vi "File_Module.vi"(7 "Command":T2, 8 "error in (no error)":errorcluster, 9 "DATOS":T1={"TIEMPO"=1.0, "sFSET1"=1.0, "sFLUJO1"=1.0, "sFSET2"=0.0, "sFLUJO2"=0.0, "sFSET3"=0.0, "sFLUJO3"=0.0, "sFSET4"=0.0, "sFLUJO4"=0.0, "TSET_SUP"=0.0, "TEMP_SUP"=0.0, "TSET_INF"=0.0, "TEMP_INF"=0.0, "TSET_CINTA"=0.0, "T_CINTA"=0.0, "TSET_EXTRA"=0.0, "T_EXTRA"=0.0, "TEMP_TB"=0.0, "PESO_TB"=0.0, "POSICION"=0.0, "V_VAPOR"=0.0, "fFSET1"=0.0, "fFLUJO1"=0.0, "fFSET2"=0.0, "fFLUJO2"=0.0, "fFSET3"=0.0, "fFLUJO3"=0.0, "fFSET4"=0.0, "fFLUJO4"=0.0} {"fFSET4" format="%.2g"; "fFSET3" format="%.2g"; "fFSET2" format="%.2g"; "fFSET1" format="%.2g"; "fFLUJO4" format="%.2g"; "fFLUJO2" format="%.2g"; "fFLUJO1" format="%.2g"; "fFLUJO3" format="%.2g"; "T_EXTRA" format="%.2g"; "TSET_EXTRA" format="%.2g"; "T_CINTA" format="%.2g"; "TSET_CINTA" format="%.2g"; "sFSET4" format="%.2g"; "POSICION" format="%.2g"; "TEMP_SUP" format="%.2g"; "TSET_SUP" format="%.2g"; "PESO_TB" format="%.2g"; "TEMP_TB" format="%.2g"; "TEMP_INF" format="%.2g"; "sFSET3" format="%.2g"; "sFSET2" format="%.2g"; "sFSET1" format="%.2g"; "V_VAPOR" format="%.2g"; "sFLUJO4" format="%.2g"; "sFLUJO2" format="%.2g"; "sFLUJO1" format="%.2g"; "TSET_INF" format="%.2g"; "TIEMPO" format="%.2g"; "sFLUJO3" format="%.2g"}, 11 "Comments":string) -> (0 "error out":errorcluster, 2 "selected path":path)   [LabVIEW 2013]
uses:
  File_Module Control.ctl
  Controles/P2022 Datos Control.ctl
  P2022 TB INCAR GLOBALES.vi
panel:
  out "Cabeceras":string[](array[string])
  # "COMENTARIOS NO ACTUALIZADOS"
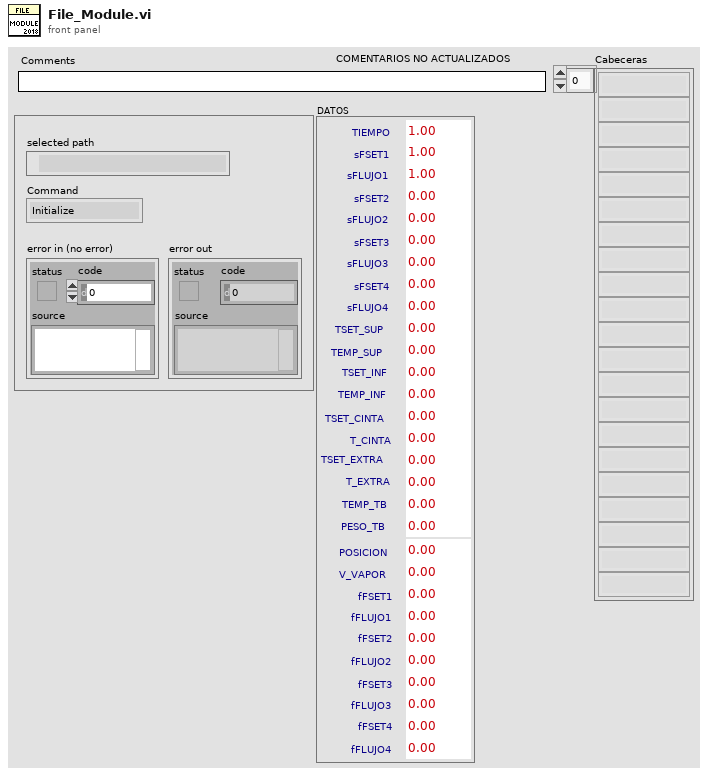
[diagram p1: front panel]
types:
  T1 = typedef "P2022 Datos Control.ctl" = cluster{"TIEMPO":dbl, "sFSET1":dbl, "sFLUJO1":dbl, "sFSET2":dbl, "sFLUJO2":dbl, "sFSET3":dbl, "sFLUJO3":dbl, "sFSET4":dbl, "sFLUJO4":dbl, "TSET_SUP":dbl, "TEMP_SUP":dbl, "TSET_INF":dbl, "TEMP_INF":dbl, "TSET_CINTA":dbl, "T_CINTA":dbl, "TSET_EXTRA":dbl, "T_EXTRA":dbl, "TEMP_TB":dbl, "PESO_TB":dbl, "POSICION":dbl, "V_VAPOR":dbl, "fFSET1":dbl, "fFLUJO1":dbl, "fFSET2":dbl, "fFLUJO2":dbl, "fFSET3":dbl, "fFLUJO3":dbl, "fFSET4":dbl, "fFLUJO4":dbl}
  T2 = typedef "File_Module Control.ctl" = enum16{"Initialize", "Save Head", "Save Data", "Shutdown"}
  T3 = enum16{"open", "replace", "create", "open or create", "replace or create", "replace or create with confirmation"}
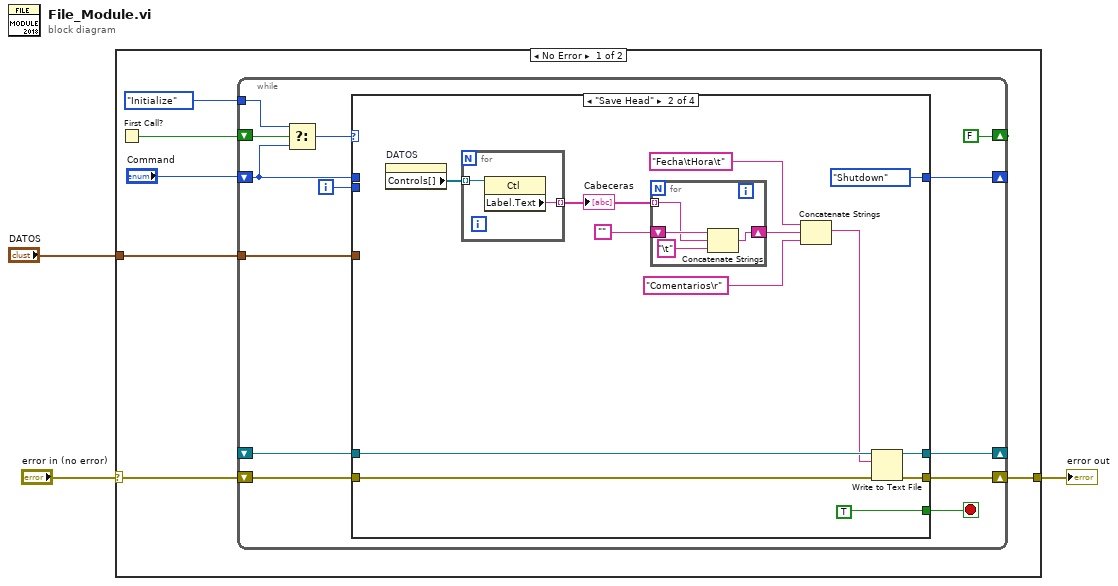
[diagram p0: block diagram]
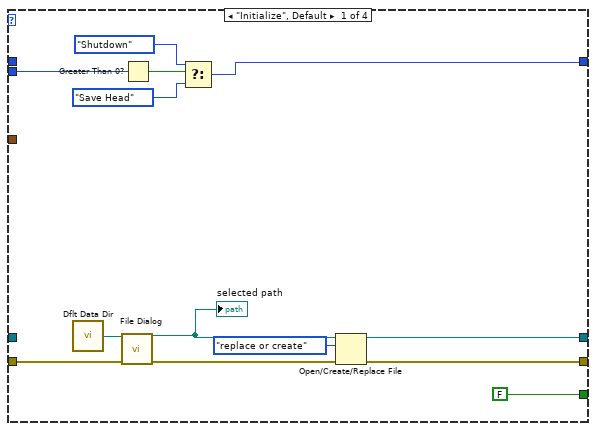
[diagram p2: hidden frame]
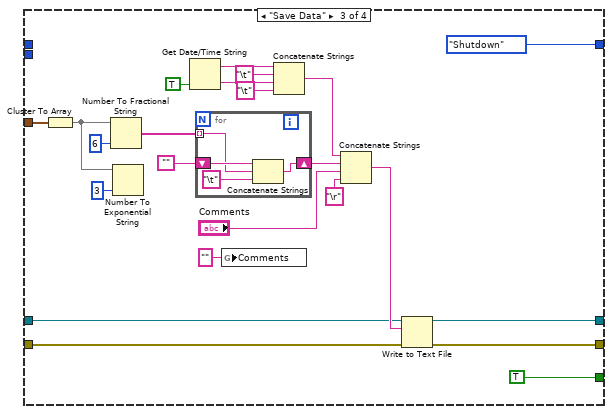
[diagram p3: hidden frame]
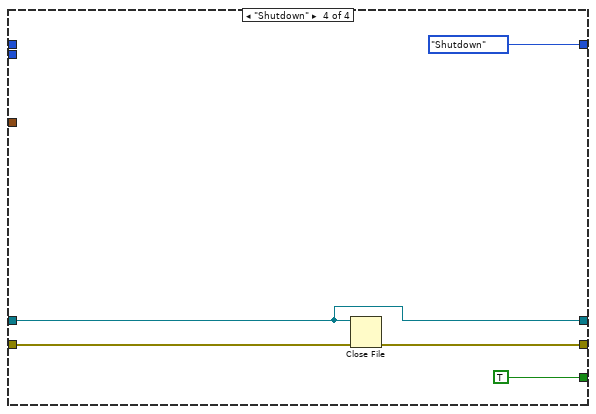
[diagram p4: hidden frame]
diagram:
  n1 = case shown="No Error" "error in (no error)" {
    selector: "error in (no error)" -> [w7 w87]
    tunnel: [w6 w87] -> w2
    tunnel: "DATOS" -> [w4 _]
    frame No Error {
      n2 = First Call?() -> (First Call?: T/F=w9:bool)
      n3 = while {
        shift-right: [w14] -> _
        shift-left: "Command" -> [w15]
        shift-right: [w17] -> w6
        shift-left: w7 -> [w18]
        shift-right: [FALSE ("First Call?: T/F")] -> _
        shift-left: w9 -> [w22]
        tunnel: File_Module_Control."Initialize" ("t") -> [w21]
        shift-right: [w11] -> _
        shift-left: _ -> [w12]
        tunnel: w4 -> [w10]
        i -> [w13]
        stop <- w19 stop-if-true
        n4 = Select(t=w21, s=w22, f=w15) -> (s? t:f=w20:T2)
        n5 = case shown="\"Save Head\"" w20 {
          tunnel: [FALSE TRUE TRUE TRUE] -> w19
          tunnel: w18 -> [w28 w44 w71 w84]
          tunnel: [w24 w43 w70 w83] -> w17
          tunnel: w15 -> [_ _ _ _]
          tunnel: [w34 File_Module_Control."Shutdown" ("t") File_Module_Control."Shutdown" File_Module_Control."Shutdown"] -> w14
          tunnel: w13 -> [w32 _ _ _]
          tunnel: w12 -> [_ w46 w67 w82]
          tunnel: [w23 w45 w69 w82] -> w11
          tunnel: w10 -> [_ _ w72 _]
          frame "Initialize", Default {
            n6 = call <vilib>:"Dflt Data Dir.vi"() -> ("App:Default Data Directory"=w29:path)
            n7 = call "File Dialog"("start path"=w29, "error in"=w28) -> ("selected path"=w26:path, "error out"=w25:errorcluster)  [unwired: 10 in, 2 out]
            "selected path" <- w26
            n8 = Greater Than 0?(x=w32) -> (x > 0?=w31:bool)
            n9 = Select(t=File_Module_Control."Shutdown", s=w31, f=File_Module_Control."Save Head" ("t")) -> (s? t:f=w34:T2)
            n10 = Open/Create/Replace File(file path (use dialog)=w26, error in=w25, operation (0:open)=T3."replace or create") -> (refnum out=w23:refnum<file>, error out=w24:errorcluster)  [unwired: 3 in, 1 out]
          }
          frame "Save Head" {
            n11 = property on="DATOS" class="Clust (strict)"() -> ("Controls[]"=w42:refnum<vi>[])  [unwired: 2 in, 2 out]
            n12 = for {
              tunnel: w42 -> [w54] mode=indexing
              tunnel: [w53] -> w38 mode=indexing
              n13 = property class="Ctl"(reference=w54) -> ("Label.Text"=w53:string)  [unwired: 1 in, 2 out]
            }
            "Cabeceras" <- w38
            n14 = for {
              tunnel: w38 -> [w51] mode=indexing
              shift-right: [w50] -> w41
              shift-left: "" -> [w52]
              n15 = Concatenate Strings(w52, w51, "\t" ("string")) -> (w50:string)
            }
            n16 = Concatenate Strings("Fecha\tHora\t" ("string"), w41, "Comentarios\r" ("string")) -> (w36:string)
            n17 = Write to Text File(file (use dialog)=w46, text=w36, error in=w44) -> (refnum out=w45:refnum<file>, error out=w43:errorcluster)  [unwired: 1 in, 1 out]
          }
          frame "Save Data" {
            n18 = Cluster To Array(cluster=w72) -> (array=w56:dbl[])
            n19 = Number To Fractional String(number=w56, precision (6)=i16 6) -> (F-format string=w55:string[])  [unwired: 2 in]
            n20 = Number To Exponential String(number=w56, precision (6)=i16 3) -> ()  [unwired: 2 in, 1 out]
            n21 = Get Date/Time String(want seconds? (F)=TRUE) -> (date string=w63:string, time string=w62:string)  [unwired: 2 in]
            n22 = for {
              tunnel: w55 -> [w80] mode=indexing
              shift-right: [w79] -> w75
              shift-left: "" -> [w81]
              n23 = Concatenate Strings(w81, w80, "\t" ("string")) -> (w79:string)
            }
            n24 = global write "P2022 TB INCAR GLOBALES.vi" "Comments"("" ("Comments")) -> ()
            n25 = Concatenate Strings(w63, "\t" ("string"), w62, "\t" ("string")) -> (w66:string)
            n26 = Concatenate Strings(w66, w75, "Comments", "\r" ("string")) -> (w68:string)
            n27 = Write to Text File(file (use dialog)=w67, text=w68, error in=w71) -> (refnum out=w69:refnum<file>, error out=w70:errorcluster)  [unwired: 1 in, 1 out]
          }
          frame "Shutdown" {
            n28 = Close File(refnum=w82, error in=w84) -> (error out=w83:errorcluster)  [unwired: 1 out]
          }
        }
      }
    }
    frame Error {
    }
  }
  "error out" <- w2
